vi "TAB_CONTROL.vi"() -> ()   [LabVIEW 2021]
panel:
  in  "Gate_control":dbl(knob) scale=0.0..100.0
  in  "Button":bool
  in  "Tab Control":enum32{"Lights", "gate"}(tab)
  out "LED":bool
  out "Gate":u8(slide) scale=0.0..100.0
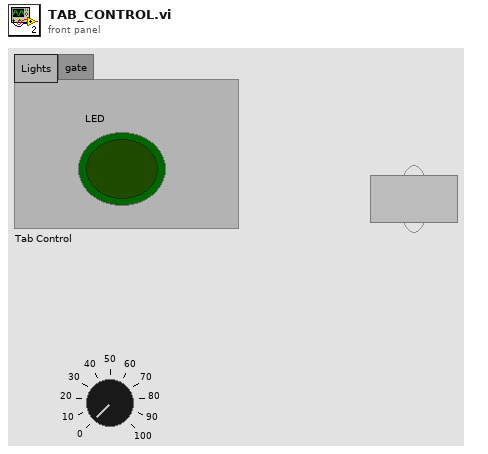
[diagram p1: front panel]
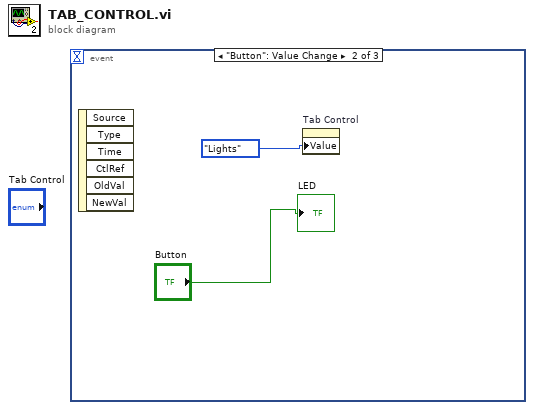
[diagram p0: block diagram]
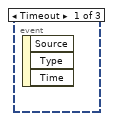
[diagram p2: hidden frame]
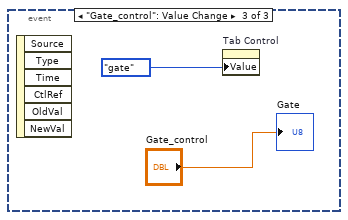
[diagram p3: hidden frame]
diagram:
  n1 = event shown="[1] \"Button\": Value Change" {
    selector: _ -> [_ _ _]
    dyn-events: _ -> [_ _ _]
    timeout: _ -> [_ _ _]
    event Timeout {
      n2 = event-data() -> ()  [unwired: 1 in, 3 out]
    }
    event "Button": Value Change {
      n3 = event-data() -> ()  [unwired: 1 in, 6 out]
      n4 = property on="Tab Control" class="TabCtl (strict)"("Value"=enum32{"Lights", "gate"}."Lights" ("Tab Control")) -> ()  [unwired: 2 in, 2 out]
      "LED" <- "Button"
    }
    event "Gate_control": Value Change {
      n5 = event-data() -> ()  [unwired: 1 in, 6 out]
      n6 = property on="Tab Control" class="TabCtl (strict)"("Value"=enum32{"Lights", "gate"}."gate" ("Tab Control")) -> ()  [unwired: 2 in, 2 out]
      "Gate" <- "Gate_control"
    }
  }
